vi "State_Machine.vi"(8 "error in (no error)":errorcluster caption="entrée d'erreur (pas d'erreur)", 11 "Get_Voltage en entrée":refnum<class "Wait_Frame_ERP1.lvclass">) -> (0 "error out":errorcluster caption="sortie d'erreur", 2 "Json_String":string, 3 "Get_Voltage en sortie":refnum<class "Wait_Frame_ERP1.lvclass">)   [LabVIEW 2020, in "Library Test.lvlib" / "Wait_Frame_ERP1.lvclass"]
uses:
  Wait_Frame_ERP1.lvclass
  C:/Users/ngarcin/OneDrive - Altyor/Standard TB/Suite TB45/Class/Test/Test (Default)/Test (Default).lvclass
  Commun VI/TypeDef/Variable Printable.ctl
  Commun VI/Library Commun.lvlib
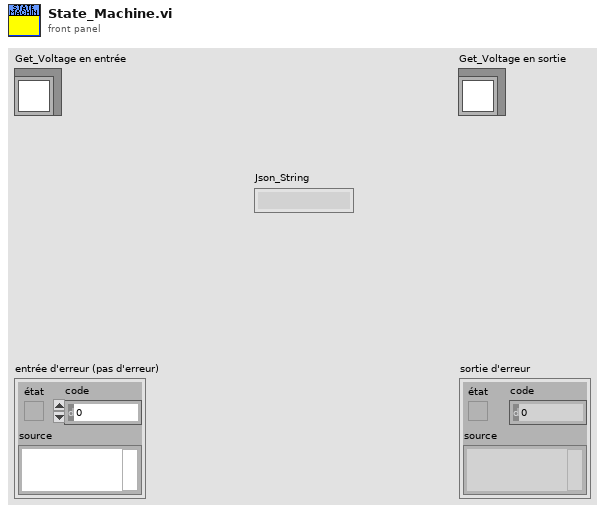
[diagram p1: front panel]
types:
  T1 = typedef "Variable Printable.ctl" = string
  T2 = enum16{"Get Variable", "Get All Variables", "Set Variable", "Delete Variable", "Delete All Variable"}
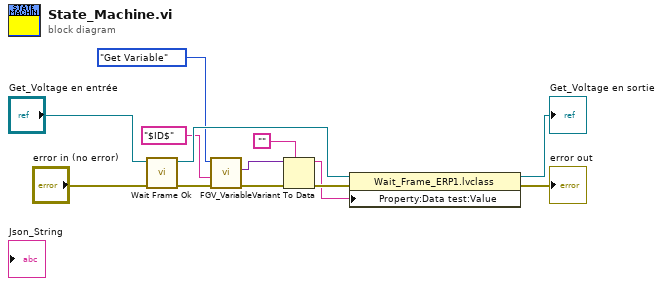
[diagram p0: block diagram]
diagram:
  n1 = call-dynamic "Wait Frame Ok.vi"("entrée d'erreur (pas d'erreur)"="error in (no error)", "Wait_Frame_ERP1 en entrée"="Get_Voltage en entrée") -> ("sortie d'erreur"=w8:errorcluster, "Wait_Frame_ERP1 en sortie"=w9:refnum<class "Wait_Frame_ERP1.lvclass">)  [unwired: 8 in]
  n2 = call "FGV_Variable.vi"("error in (no error)"=w8, "Variable"=T1 "$ID$", "Function"=T2."Get Variable") -> ("error out"=w5:errorcluster, "Data Out"=w3:variant)  [unwired: 6 in, 1 out]
  n3 = Variant To Data(error in=w5, type="", Variant=w3) -> (data=w1:string, error out=w4:errorcluster)
  n4 = property class="Wait_Frame_ERP1.lvclass"(reference=w9, error in=w4, "Property:Data test:Value"=w1) -> (reference out=→"Get_Voltage en sortie":refnum<class "Wait_Frame_ERP1.lvclass">, error out=→"error out":errorcluster)
